vi "SetCurrentLang.vi"(0 "Lang":u16(ring) caption="Language" items=["ENGLISH", "简体中文", "Dutch"]) -> ()   [LabVIEW 2010]
uses:
  <vilib>/Utility/config.llb/Write Key (U32).vi
  <vilib>/Utility/config.llb/NI_LVConfig.lvlib
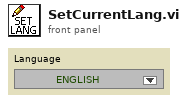
[diagram p1: front panel]
types:
  T1 = typedef "NI_LVConfig.lvlib/Config Data RefNum.ctl" = refnum<k1>
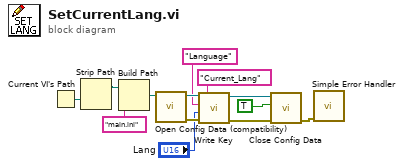
[diagram p0: block diagram]
diagram:
  n1 = Current VI's Path() -> (path=w13:path)
  n2 = Strip Path(path=w13) -> (stripped path=w12:path)  [unwired: 1 out]
  n3 = Build Path(base path=w12, name or relative path="main.ini") -> (appended path=w11:path)
  n4 = call <vilib>:"Open Config Data (compatibility).vi"("configuration file path"=w11) -> ("error out"=w7:errorcluster, "refnum"=w8:T1)  [unwired: 8 in, 1 out]
  n5 = call-poly <vilib>:"Write Key.vi"("section"="Current_Lang", "error in (no error)"=w7, "value"="Lang", "key"="Language", "refnum"=w8) -> ("error out"=w1:errorcluster, "refnum out"=w2:T1)  [unwired: 5 out]
  n6 = call <vilib>:"Close Config Data.vi"("error in (no error)"=w1, "write file if changed (T)"=TRUE ("write configuration file? (T)"), "refnum"=w2) -> ("error out"=w10:errorcluster)  [unwired: 8 out]
  n7 = call <vilib>:"Simple Error Handler.vi"("error in (no error)"=w10) -> ()  [unwired: 1 in, 8 out]
